vi "1D Gaussian Fitting.vi"(0 "X Values":dbl[](array[numeric]), 7 "Y Values":dbl[](array[numeric])) -> (4 "X Values Out":dbl[](array[numeric]), 8 "Y Values Out":dbl[](array[numeric]), 15 "Best Fit Parameters":dbl[](array[numeric]))   [LabVIEW 2016]
doc: "Fit (x, y) data with 1D Gaussian. Best fit parameter array is as follows:\n\n1. Amplitude\n2. Center Position\n3. Width\n4. Offset"
uses:
  <vilib>/Analysis/NI_AALPro.lvlib
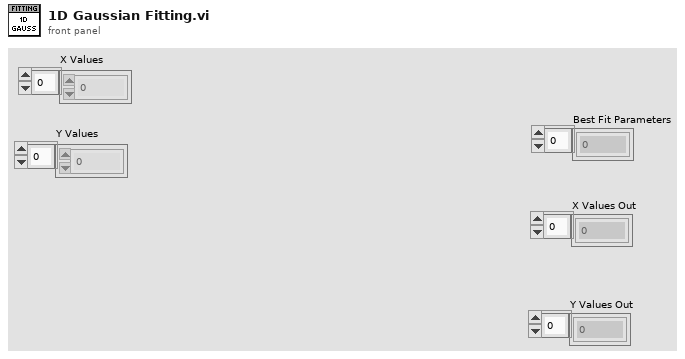
[diagram p1: front panel]
types:
  T1 = cluster{"initial amplitude":dbl, "initial center":dbl, "initial standard deviation":dbl, "offset":dbl}
  T2 = cluster{"amp min":dbl, "amp max":dbl, "center min":dbl, "center max":dbl, "deviation min":dbl, "deviation max":dbl, "offset min":dbl, "offset max":dbl}
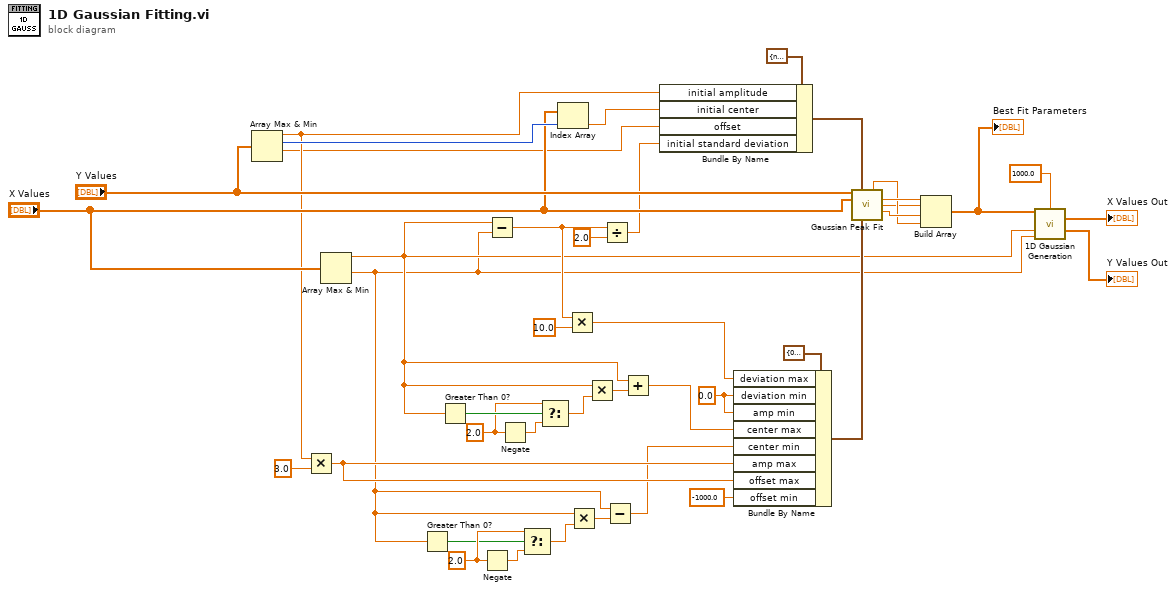
[diagram p0: block diagram]
diagram:
  w8 = 2.0 ("y")
  w13 = 2.0 ("y")
  w20 = 0.0 ("amp min")
  n1 = Array Max & Min(array="Y Values") -> (max value=w22:dbl, max index (indices)=w34:i32, min value=w21:dbl)  [unwired: 1 out]
  n2 = Multiply(x=w22, y=3.0 ("x")) -> (x*y=w19:dbl)
  n3 = Array Max & Min(array="X Values") -> (max value=w11:dbl, min value=w1:dbl)  [unwired: 2 out]
  n4 = Greater Than 0?(x=w1) -> (x > 0?=w6:bool)
  n5 = Greater Than 0?(x=w11) -> (x > 0?=w15:bool)
  n6 = Negate(x=w8) -> (-x=w9:dbl)
  n7 = Subtract(x=w11, y=w1) -> (x-y=w25:dbl)
  n8 = Negate(x=w13) -> (-x=w12:dbl)
  n9 = Select(t=w8, s=w6, f=w9) -> (s? t:f=w7:dbl)
  n10 = Select(t=w13, s=w15, f=w12) -> (s? t:f=w14:dbl)
  n11 = Index Array(array="X Values", index=w34) -> (element=w28:dbl)
  n12 = Multiply(x=w25, y=10.0) -> (x*y=w18:dbl)
  n13 = Multiply(x=w1, y=w7) -> (x*y=w5:dbl)
  n14 = Multiply(x=w11, y=w14) -> (x*y=w16:dbl)
  n15 = Divide(x=w25, y=2.0) -> (x/y=w27:dbl)
  n16 = Subtract(x=w1, y=w5) -> (x-y=w4:dbl)
  n17 = Add(x=w11, y=w16) -> (x+y=w10:dbl)
  n18 = Bundle By Name(cluster=T1 {"initial amplitude"=nan, "initial center"=nan, "initial standard deviation"=nan, "offset"=nan} ("initial guess"), "initial amplitude"=w22, "initial center"=w28, "offset"=w21, "initial standard deviation"=w27) -> (w26:T1)
  n19 = Bundle By Name(cluster=T2 {"amp min"=0.0, "amp max"=100000.0, "center min"=-100.0, "center max"=100.0, "deviation min"=0.0, "deviation max"=1000.0, "offset min"=0.0, "offset max"=1000.0} ("parameter bounds"), "deviation max"=w18, "deviation min"=w20, "amp min"=w20, "center max"=w10, "center min"=w4, "amp max"=w19, "offset max"=w19, "offset min"=-1000.0) -> (w32:T2)
  n20 = call <vilib>:"Gaussian Peak Fit.vi"("Y"="Y Values", "initial guess"=w26, "X"="X Values", "parameter bounds"=w32) -> ("offset"=w39:dbl, "amplitude"=w41:dbl, "center"=w36:dbl, "standard deviation"=w40:dbl)  [unwired: 5 in, 3 out]
  n21 = Build Array(w41, w36, w40, w39) -> (w38:dbl[])
  "Best Fit Parameters" <- w38
  n22 = call "1D Gaussian Generation.vi"("Parameters In"=w38, "Number of Points"=1000.0, "Max X Value"=w11, "Min X Value"=w1) -> ("X Values"=→"X Values Out":dbl[], "Y Values"=→"Y Values Out":dbl[])  [unwired: 10 in]
